vi "PicohrdlChannelScaling.vi"(6 "Max_adc":i32=32767, 7 "Channel N":cluster{"N":bool, "Ch N":i16}={"N"=TRUE, "Ch N"=0} {"Ch N" items=["2500mV", "1225mV", "625mV", "313mV", "156mV", "78mV", "39mV"]}, 10 "DataIn":i32[](array[numeric])) -> (2 "DataOut":dbl[](array[numeric]))   [LabVIEW 2010]
doc: "Scales ADC vaules from unit to mV."
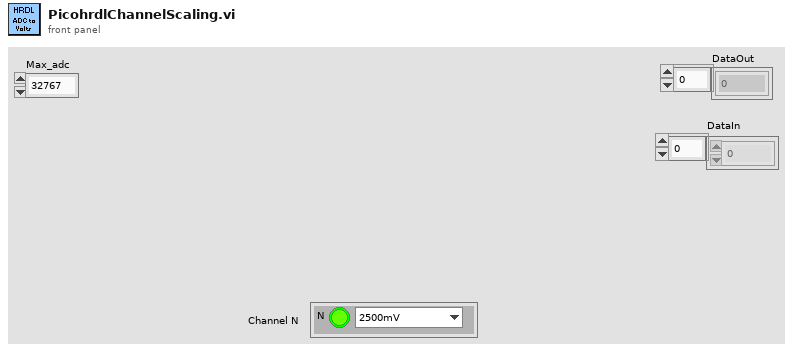
[diagram p1: front panel]
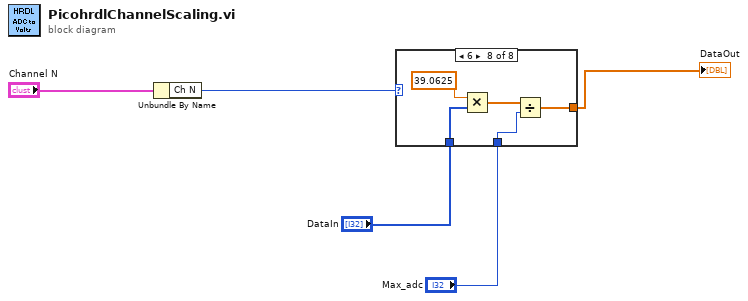
[diagram p0: block diagram]
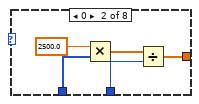
[diagram p3: hidden frame]
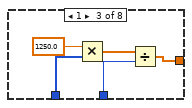
[diagram p4: hidden frame]
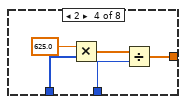
[diagram p5: hidden frame]
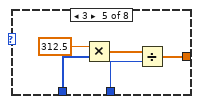
[diagram p6: hidden frame]
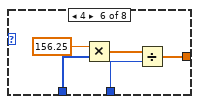
[diagram p7: hidden frame]
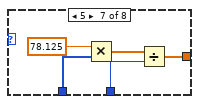
[diagram p8: hidden frame]
diagram:
  n1 = Unbundle By Name("Channel N") -> ("Ch N"=w1:i16)
  n2 = case shown="6" w1 {
    tunnel: [w6 w9 w13 w19 w24 w29 w34 w38] -> w5
    tunnel: "DataIn" -> [w6 w7 w14 w18 w23 w28 w33 w39]
    tunnel: "Max_adc" -> [_ w8 w12 w17 w22 w27 w32 w37]
    frame Default {
    }
    frame 0 {
      n3 = Multiply(x=2500.0, y=w7) -> (x*y=w10:dbl[])
      n4 = Divide(x=w10, y=w8) -> (x/y=w9:dbl[])
    }
    frame 1 {
      n5 = Multiply(x=1250.0, y=w14) -> (x*y=w16:dbl[])
      n6 = Divide(x=w16, y=w12) -> (x/y=w13:dbl[])
    }
    frame 2 {
      n7 = Multiply(x=625.0, y=w18) -> (x*y=w20:dbl[])
      n8 = Divide(x=w20, y=w17) -> (x/y=w19:dbl[])
    }
    frame 3 {
      n9 = Multiply(x=312.5, y=w23) -> (x*y=w25:dbl[])
      n10 = Divide(x=w25, y=w22) -> (x/y=w24:dbl[])
    }
    frame 4 {
      n11 = Multiply(x=156.25, y=w28) -> (x*y=w31:dbl[])
      n12 = Divide(x=w31, y=w27) -> (x/y=w29:dbl[])
    }
    frame 5 {
      n13 = Multiply(x=78.125, y=w33) -> (x*y=w36:dbl[])
      n14 = Divide(x=w36, y=w32) -> (x/y=w34:dbl[])
    }
    frame 6 {
      n15 = Multiply(x=39.0625, y=w39) -> (x*y=w41:dbl[])
      n16 = Divide(x=w41, y=w37) -> (x/y=w38:dbl[])
    }
  }
  "DataOut" <- w5
